vi "2D Maze to 1D.vi"(11 "Maze (0: Empty, -1: Enemy. >0: Teammate":i32[][](array[numeric])) -> (3 "1D Maze":i32[](array[numeric]))   [LabVIEW 2015]
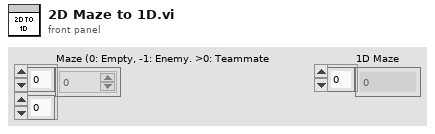
[diagram p1: front panel]
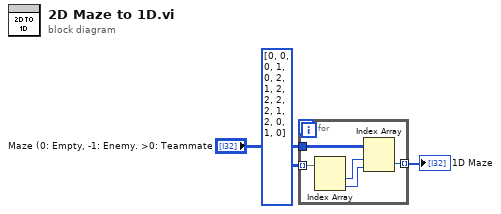
[diagram p0: block diagram]
diagram:
  n1 = for {
    tunnel: "Maze (0: Empty, -1: Enemy. >0: Teammate" -> [w8]
    tunnel: i32[][] [[0, 0], [0, 1], [0, 2], [1, 2], [2, 2], [2, 1], [2, 0], [1, 0]] -> [w7] mode=indexing
    tunnel: [w4] -> w3 mode=indexing
    n2 = Index Array(array=w7) -> (element #1=w6:i32, element #2=w5:i32)  [unwired: 2 in]
    n3 = Index Array(array=w8, index (row)=w6, index (col)=w5) -> (element=w4:i32)
  }
  "1D Maze" <- w3
